vi "save_config_v4_svi.vi"(0 "Refnum VISA en entrée":refnum<visa-resource-name>, 1 "Camera infos":string, 2 "Config Directory":path, 3 "USED_LEDS":bool[][](array[boolean]), 4 "STAGE_SPEED":dbl, 5 "Non_fluidics":u32, 6 "XYPOS":T1, 7 "Nstart_fluidics":u32, 8 "ROMODE":u32, 9 "NSCAN":u32, 10 "BIN":u16, 11 "USED_FILTERS":u8[](array[numeric]), 12 "EXPT":dbl, 13 "BETWEEN_SCAN":u32, 14 "config Name":string, 15 "useFLUIDICS":bool, 16 "SOFT_VERSION":string, 17 "MIN. SCAN duration":dbl, 18 "Noff_fluidics":u32, 19 "BETWEEN_PAT":u32, 20 "NPAT":u32, 21 "Noff_laser":u32, 22 "Non_laser":u32, 23 "Nstart_laser":u32, 24 "SHOOT duration":dbl, 25 "shoot_at_SCAN":u32, 26 "isSINGLEshoot":bool, 27 "useLASER":bool) -> ()   [LabVIEW 2013]
uses:
  <vilib>/Analysis/Matrix/Datatypes/RealMatrix.ctl
  <vilib>/Analysis/Matrix/NI_Matrix.lvlib
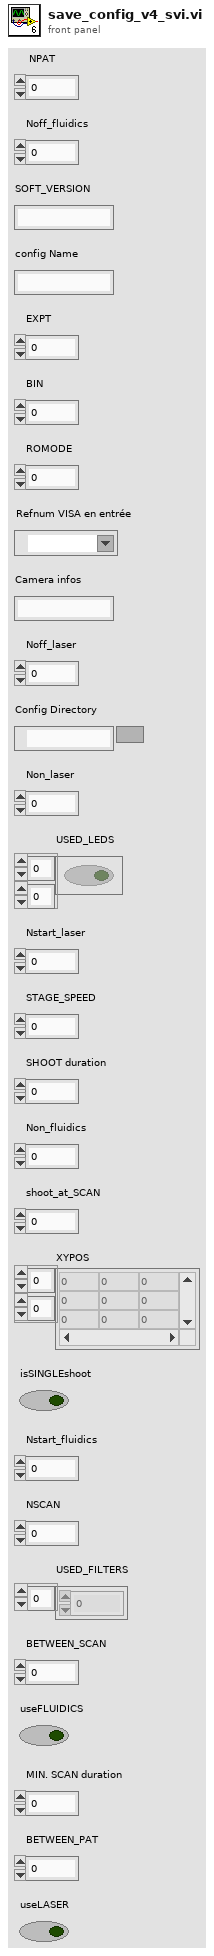
[diagram p1: front panel]
types:
  T1 = typedef "NI_Matrix.lvlib/RealMatrix.ctl" = dbl[][]
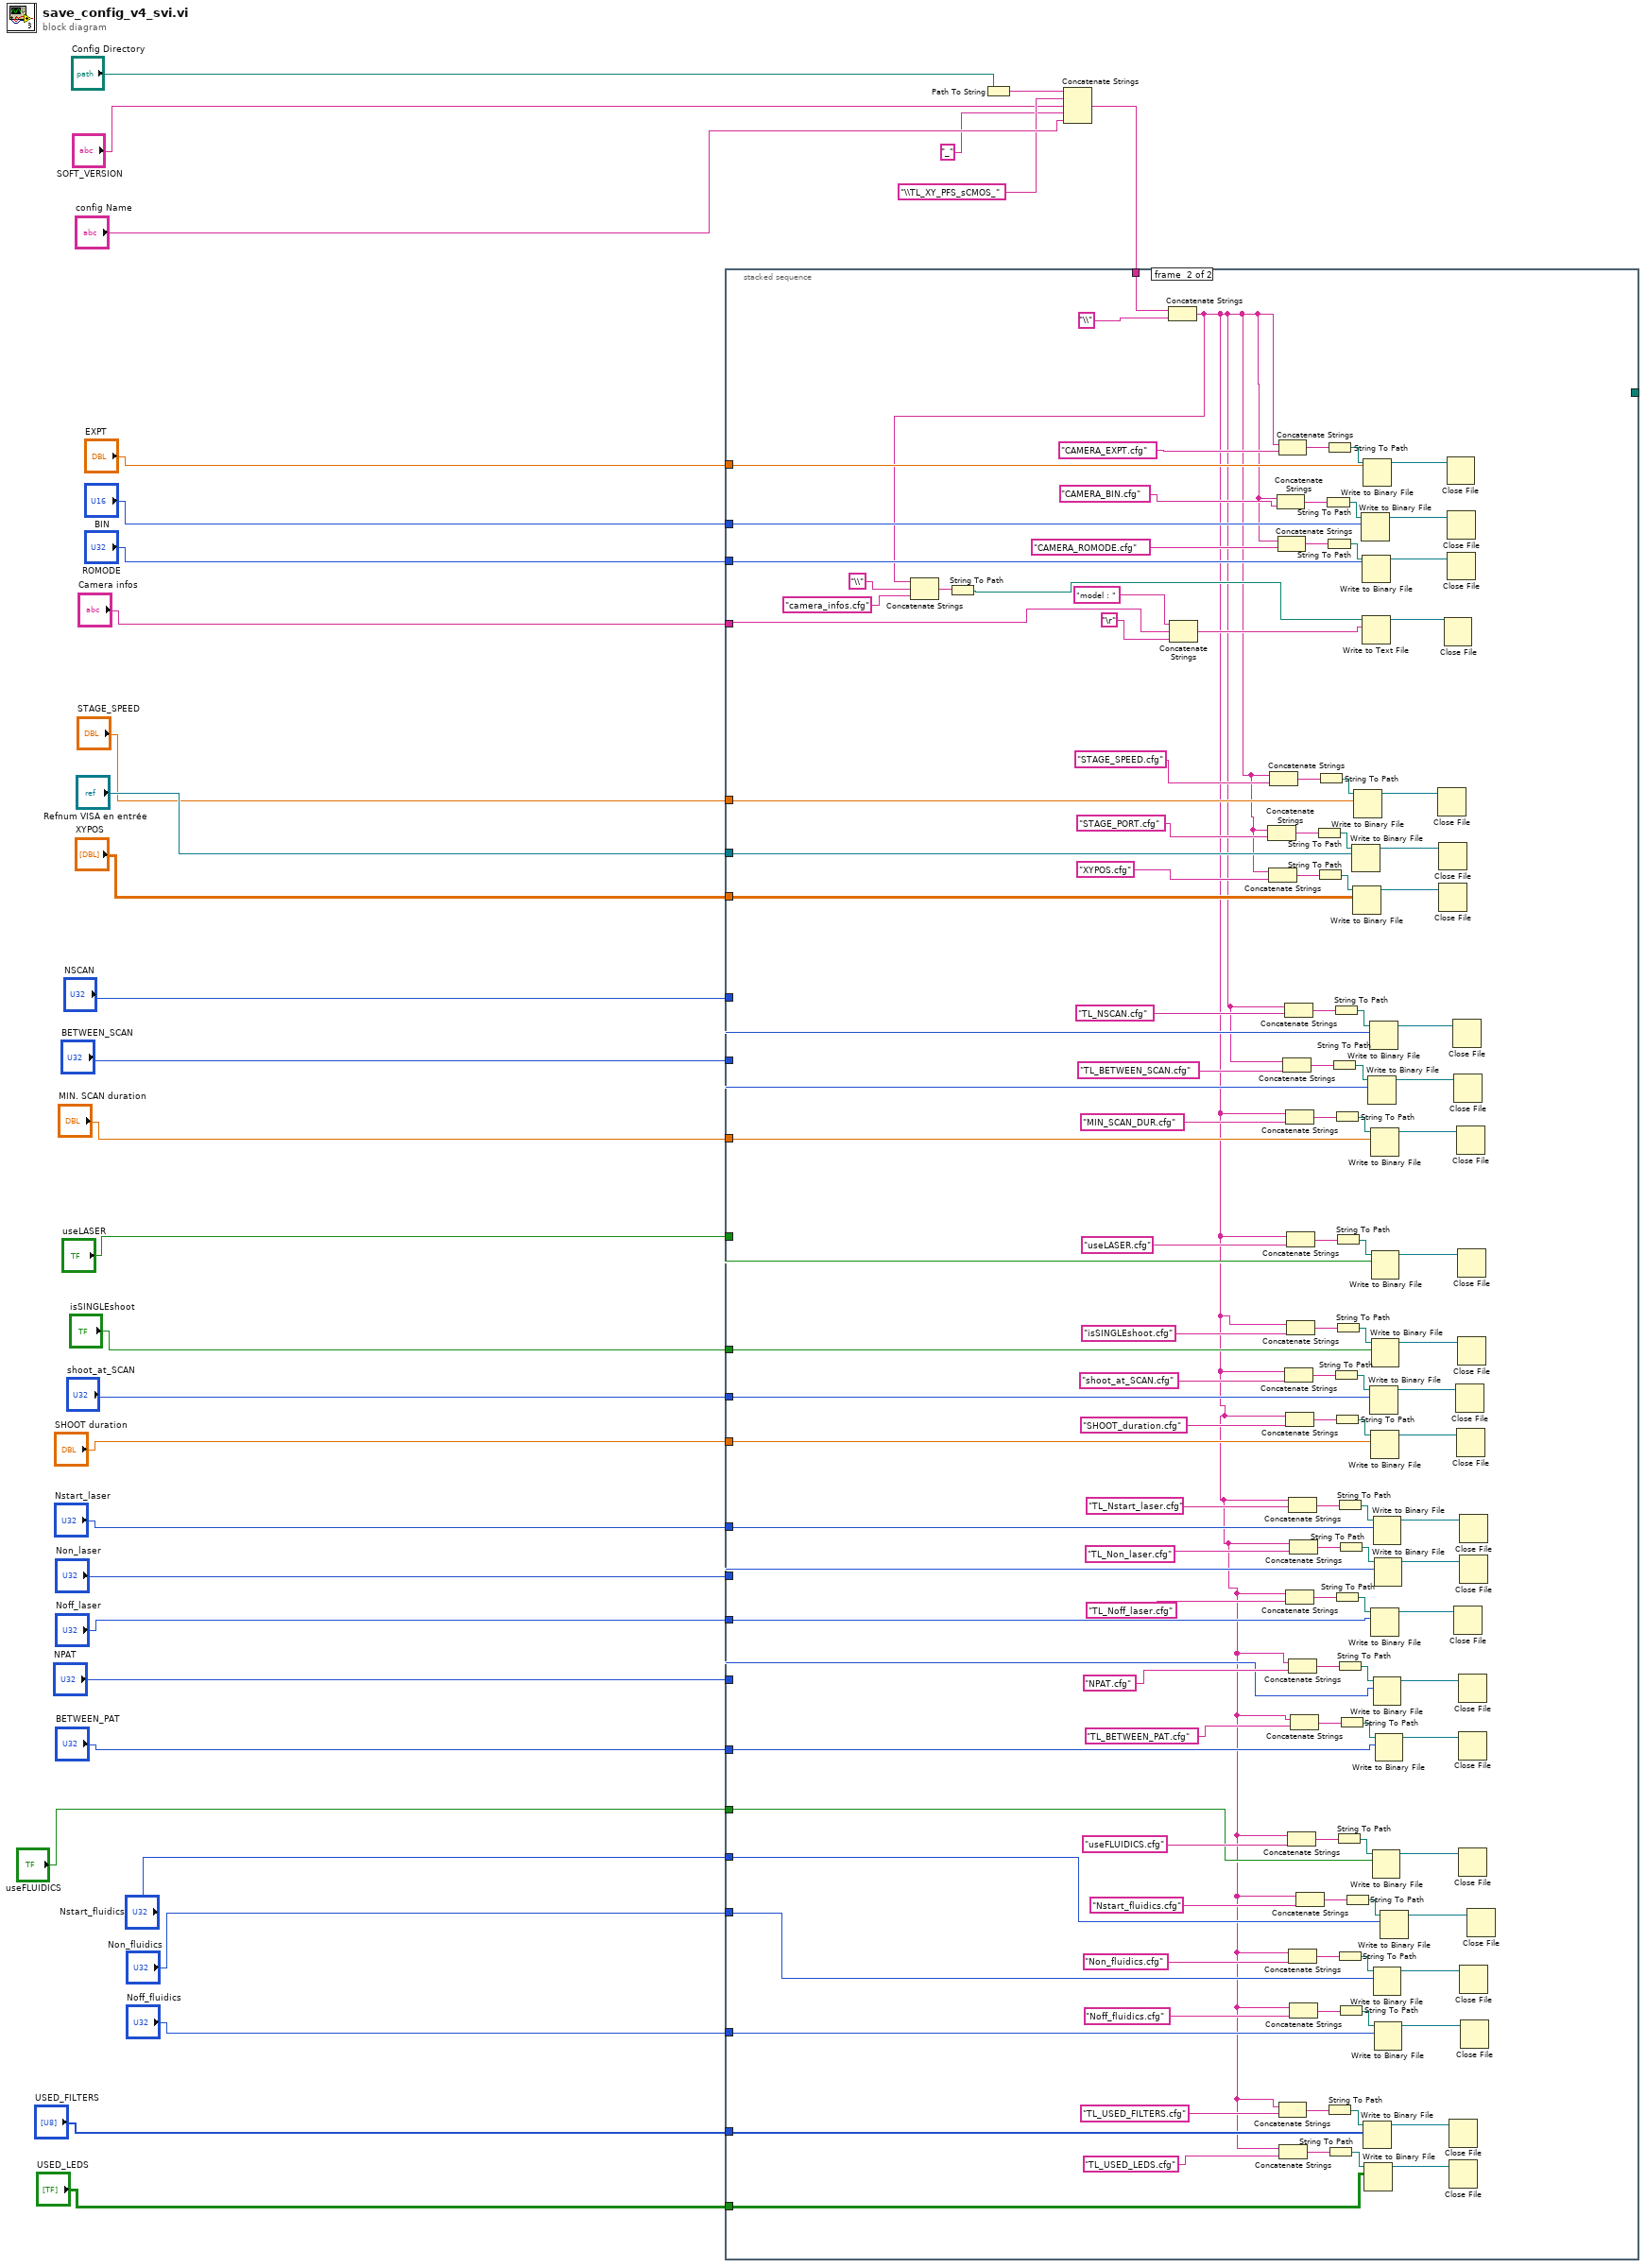
[diagram p0: block diagram]
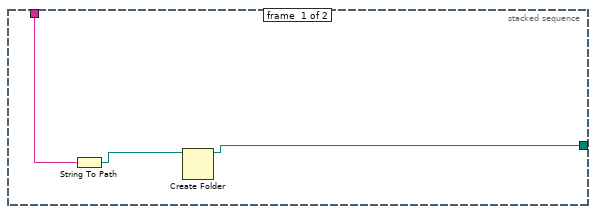
[diagram p2: hidden frame]
diagram:
  n1 = Path To String(path="Config Directory") -> (string=w6:string)
  n2 = Concatenate Strings(w6, "\\TL_XY_PFS_sCMOS_", "SOFT_VERSION", "_", "config Name") -> (w1:string)
  n3 = stacked-sequence {
    tunnel: w1 -> [w34 w100]
    tunnel: [w33 _] -> _
    tunnel: "EXPT" -> [_ w61]
    tunnel: "BIN" -> [_ w60]
    tunnel: "ROMODE" -> [_ w59]
    tunnel: "Camera infos" -> [_ w58]
    tunnel: "STAGE_SPEED" -> [_ w57]
    tunnel: "Refnum VISA en entrée" -> [_ w56]
    tunnel: "XYPOS" -> [_ w55]
    tunnel: "NSCAN" -> [_ w54]
    tunnel: "BETWEEN_SCAN" -> [_ w53]
    tunnel: "MIN. SCAN duration" -> [_ w52]
    tunnel: "useLASER" -> [_ w51]
    tunnel: "isSINGLEshoot" -> [_ w50]
    tunnel: "shoot_at_SCAN" -> [_ w49]
    tunnel: "SHOOT duration" -> [_ w48]
    tunnel: "Nstart_laser" -> [_ w47]
    tunnel: "Non_laser" -> [_ w46]
    tunnel: "Noff_laser" -> [_ w45]
    tunnel: "NPAT" -> [_ w44]
    tunnel: "BETWEEN_PAT" -> [_ w43]
    tunnel: "Noff_fluidics" -> [_ w42]
    tunnel: "Non_fluidics" -> [_ w41]
    tunnel: "Nstart_fluidics" -> [_ w40]
    tunnel: "useFLUIDICS" -> [_ w39]
    tunnel: "USED_FILTERS" -> [_ w38]
    tunnel: "USED_LEDS" -> [_ w37]
    frame #0 {
      n4 = String To Path(string=w34) -> (path=w35:path)
      n5 = Create Folder(path (use dialog)=w35) -> (created path=w33:path)  [unwired: 2 in, 2 out]
    }
    frame #1 {
      n6 = Concatenate Strings(w100, "\\") -> (w36:string)
      n7 = Concatenate Strings(w36, "\\", "camera_infos.cfg") -> (w164:string)
      n8 = String To Path(string=w164) -> (path=w167:path)
      n9 = Concatenate Strings("model : ", w58, "\r") -> (w111:string)
      n10 = Concatenate Strings(w36, "STAGE_PORT.cfg") -> (w117:string)
      n11 = Concatenate Strings(w36, "XYPOS.cfg") -> (w118:string)
      n12 = Concatenate Strings(w36, "STAGE_SPEED.cfg") -> (w116:string)
      n13 = Concatenate Strings(w36, "CAMERA_BIN.cfg") -> (w104:string)
      n14 = Concatenate Strings(w36, "CAMERA_ROMODE.cfg") -> (w108:string)
      n15 = Concatenate Strings(w36, "CAMERA_EXPT.cfg") -> (w103:string)
      n16 = Concatenate Strings(w36, "TL_USED_FILTERS.cfg") -> (w147:string)
      n17 = Concatenate Strings(w36, "TL_USED_LEDS.cfg") -> (w148:string)
      n18 = Concatenate Strings(w36, "TL_BETWEEN_SCAN.cfg") -> (w129:string)
      n19 = Concatenate Strings(w36, "TL_NSCAN.cfg") -> (w128:string)
      n20 = Concatenate Strings(w36, "shoot_at_SCAN.cfg") -> (w82:string)
      n21 = Concatenate Strings(w36, "MIN_SCAN_DUR.cfg") -> (w94:string)
      n22 = Concatenate Strings(w36, "SHOOT_duration.cfg") -> (w78:string)
      n23 = Concatenate Strings(w36, "TL_Noff_laser.cfg") -> (w146:string)
      n24 = Concatenate Strings(w36, "useLASER.cfg") -> (w90:string)
      n25 = Concatenate Strings(w36, "isSINGLEshoot.cfg") -> (w86:string)
      n26 = Concatenate Strings(w36, "useFLUIDICS.cfg") -> (w74:string)
      n27 = Concatenate Strings(w36, "TL_Nstart_laser.cfg") -> (w138:string)
      n28 = Concatenate Strings(w36, "NPAT.cfg") -> (w130:string)
      n29 = Concatenate Strings(w36, "Non_fluidics.cfg") -> (w66:string)
      n30 = Concatenate Strings(w36, "TL_Non_laser.cfg") -> (w139:string)
      n31 = Concatenate Strings(w36, "Noff_fluidics.cfg") -> (w62:string)
      n32 = Concatenate Strings(w36, "TL_BETWEEN_PAT.cfg") -> (w137:string)
      n33 = Concatenate Strings(w36, "Nstart_fluidics.cfg") -> (w70:string)
      n34 = String To Path(string=w117) -> (path=w120:path)
      n35 = String To Path(string=w118) -> (path=w121:path)
      n36 = String To Path(string=w116) -> (path=w119:path)
      n37 = String To Path(string=w104) -> (path=w105:path)
      n38 = String To Path(string=w108) -> (path=w109:path)
      n39 = String To Path(string=w103) -> (path=w101:path)
      n40 = String To Path(string=w147) -> (path=w150:path)
      n41 = String To Path(string=w148) -> (path=w151:path)
      n42 = String To Path(string=w129) -> (path=w132:path)
      n43 = String To Path(string=w128) -> (path=w131:path)
      n44 = String To Path(string=w82) -> (path=w83:path)
      n45 = String To Path(string=w94) -> (path=w95:path)
      n46 = String To Path(string=w78) -> (path=w79:path)
      n47 = String To Path(string=w146) -> (path=w149:path)
      n48 = String To Path(string=w90) -> (path=w91:path)
      n49 = String To Path(string=w86) -> (path=w87:path)
      n50 = String To Path(string=w74) -> (path=w75:path)
      n51 = String To Path(string=w138) -> (path=w141:path)
      n52 = String To Path(string=w130) -> (path=w133:path)
      n53 = String To Path(string=w66) -> (path=w67:path)
      n54 = String To Path(string=w139) -> (path=w142:path)
      n55 = String To Path(string=w62) -> (path=w63:path)
      n56 = String To Path(string=w137) -> (path=w140:path)
      n57 = String To Path(string=w70) -> (path=w71:path)
      n58 = Write to Binary File(file (use dialog)=w120, data=w56) -> (refnum out=w123:refnum<file>)  [unwired: 4 in, 2 out]
      n59 = Write to Binary File(file (use dialog)=w121, data=w55) -> (refnum out=w124:refnum<file>)  [unwired: 4 in, 2 out]
      n60 = Write to Binary File(file (use dialog)=w119, data=w57) -> (refnum out=w122:refnum<file>)  [unwired: 4 in, 2 out]
      n61 = Write to Binary File(file (use dialog)=w105, data=w60) -> (refnum out=w113:refnum<file>)  [unwired: 4 in, 2 out]
      n62 = Write to Binary File(file (use dialog)=w109, data=w59) -> (refnum out=w114:refnum<file>)  [unwired: 4 in, 2 out]
      n63 = Write to Text File(file (use dialog)=w167, text=w111) -> (refnum out=w115:refnum<file>)  [unwired: 2 in, 2 out]
      n64 = Write to Binary File(file (use dialog)=w101, data=w61) -> (refnum out=w112:refnum<file>)  [unwired: 4 in, 2 out]
      n65 = Write to Binary File(file (use dialog)=w150, data=w38) -> (refnum out=w153:refnum<file>)  [unwired: 4 in, 2 out]
      n66 = Write to Binary File(file (use dialog)=w151, data=w37) -> (refnum out=w154:refnum<file>)  [unwired: 4 in, 2 out]
      n67 = Write to Binary File(file (use dialog)=w132, data=w53) -> (refnum out=w135:refnum<file>)  [unwired: 4 in, 2 out]
      n68 = Write to Binary File(file (use dialog)=w131, data=w54) -> (refnum out=w134:refnum<file>)  [unwired: 4 in, 2 out]
      n69 = Write to Binary File(file (use dialog)=w83, data=w49) -> (refnum out=w84:refnum<file>)  [unwired: 4 in, 2 out]
      n70 = Write to Binary File(file (use dialog)=w95, data=w52) -> (refnum out=w96:refnum<file>)  [unwired: 4 in, 2 out]
      n71 = Write to Binary File(file (use dialog)=w79, data=w48) -> (refnum out=w80:refnum<file>)  [unwired: 4 in, 2 out]
      n72 = Write to Binary File(file (use dialog)=w149, data=w45) -> (refnum out=w152:refnum<file>)  [unwired: 4 in, 2 out]
      n73 = Write to Binary File(file (use dialog)=w91, data=w51) -> (refnum out=w92:refnum<file>)  [unwired: 4 in, 2 out]
      n74 = Write to Binary File(file (use dialog)=w87, data=w50) -> (refnum out=w88:refnum<file>)  [unwired: 4 in, 2 out]
      n75 = Write to Binary File(file (use dialog)=w75, data=w39) -> (refnum out=w76:refnum<file>)  [unwired: 4 in, 2 out]
      n76 = Write to Binary File(file (use dialog)=w141, data=w47) -> (refnum out=w144:refnum<file>)  [unwired: 4 in, 2 out]
      n77 = Write to Binary File(file (use dialog)=w133, data=w44) -> (refnum out=w136:refnum<file>)  [unwired: 4 in, 2 out]
      n78 = Write to Binary File(file (use dialog)=w67, data=w41) -> (refnum out=w68:refnum<file>)  [unwired: 4 in, 2 out]
      n79 = Write to Binary File(file (use dialog)=w142, data=w46) -> (refnum out=w145:refnum<file>)  [unwired: 4 in, 2 out]
      n80 = Write to Binary File(file (use dialog)=w63, data=w42) -> (refnum out=w64:refnum<file>)  [unwired: 4 in, 2 out]
      n81 = Write to Binary File(file (use dialog)=w140, data=w43) -> (refnum out=w143:refnum<file>)  [unwired: 4 in, 2 out]
      n82 = Write to Binary File(file (use dialog)=w71, data=w40) -> (refnum out=w72:refnum<file>)  [unwired: 4 in, 2 out]
      n83 = Close File(refnum=w122) -> ()  [unwired: 1 in, 2 out]
      n84 = Close File(refnum=w123) -> ()  [unwired: 1 in, 2 out]
      n85 = Close File(refnum=w124) -> ()  [unwired: 1 in, 2 out]
      n86 = Close File(refnum=w115) -> ()  [unwired: 1 in, 2 out]
      n87 = Close File(refnum=w112) -> ()  [unwired: 1 in, 2 out]
      n88 = Close File(refnum=w113) -> ()  [unwired: 1 in, 2 out]
      n89 = Close File(refnum=w114) -> ()  [unwired: 1 in, 2 out]
      n90 = Close File(refnum=w153) -> ()  [unwired: 1 in, 2 out]
      n91 = Close File(refnum=w154) -> ()  [unwired: 1 in, 2 out]
      n92 = Close File(refnum=w134) -> ()  [unwired: 1 in, 2 out]
      n93 = Close File(refnum=w135) -> ()  [unwired: 1 in, 2 out]
      n94 = Close File(refnum=w152) -> ()  [unwired: 1 in, 2 out]
      n95 = Close File(refnum=w84) -> ()  [unwired: 1 in, 2 out]
      n96 = Close File(refnum=w96) -> ()  [unwired: 1 in, 2 out]
      n97 = Close File(refnum=w80) -> ()  [unwired: 1 in, 2 out]
      n98 = Close File(refnum=w92) -> ()  [unwired: 1 in, 2 out]
      n99 = Close File(refnum=w88) -> ()  [unwired: 1 in, 2 out]
      n100 = Close File(refnum=w136) -> ()  [unwired: 1 in, 2 out]
      n101 = Close File(refnum=w143) -> ()  [unwired: 1 in, 2 out]
      n102 = Close File(refnum=w76) -> ()  [unwired: 1 in, 2 out]
      n103 = Close File(refnum=w144) -> ()  [unwired: 1 in, 2 out]
      n104 = Close File(refnum=w145) -> ()  [unwired: 1 in, 2 out]
      n105 = Close File(refnum=w68) -> ()  [unwired: 1 in, 2 out]
      n106 = Close File(refnum=w64) -> ()  [unwired: 1 in, 2 out]
      n107 = Close File(refnum=w72) -> ()  [unwired: 1 in, 2 out]
    }
  }
